vi "test_sample_and_fetch.vi"() -> ()   [LabVIEW 2013, in "varilib.lvlib"]
uses:
  varilib.lvlib
  <instrlib>/niScope/Configure/Trigger/niScope Configure Trigger Immediate.vi
panel:
  in  "status":string
  out "sampling start times":timestamp[](array[timestamp])
  in  "channels (0,1)":string[](array[string])
  in  "generate time axis (T)":bool
  in  "instrument handles":refnum<k15>[](array[refnum])
  out "error out":errorcluster
  out "no of vars in matlab file":i32
  in  "file format (mat)":T1(ring)=enum."csv - semicolon separated values"
  in  "file path and name":path=path "c:/smazat.csv"
  in  "min sample rate":dbl=15000000.0 format="%#_13p"
  in  "min record length":i32=30000000 format="%.0p"
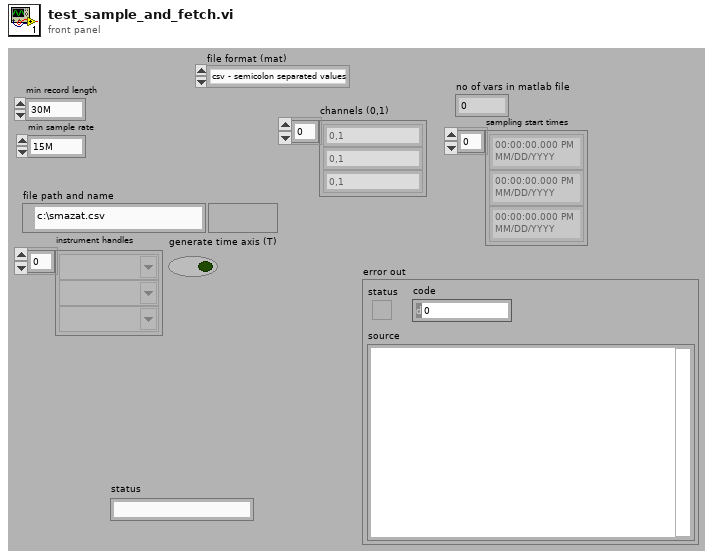
[diagram p1: front panel]
types:
  T1 = enum16{"mat - matlab binary", "csv - semicolon separated values"}
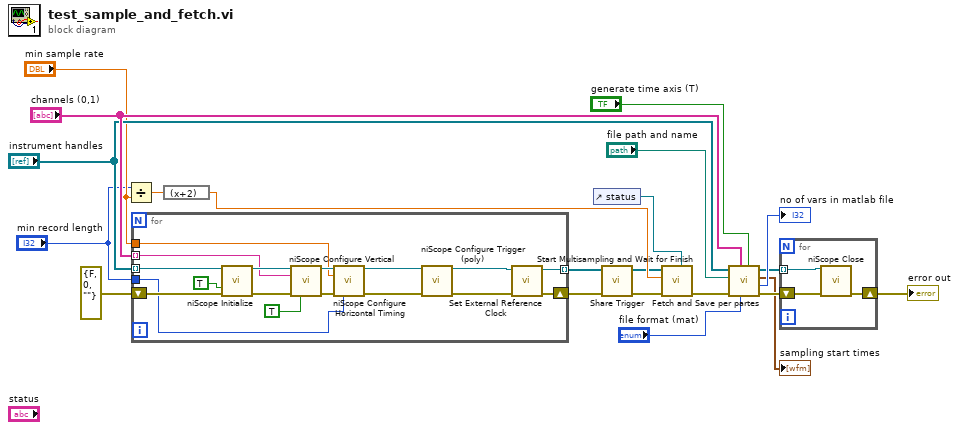
[diagram p0: block diagram]
diagram:
  n1 = Divide(x="min record length", y="min sample rate") -> (x/y=w9:dbl)
  n2 = for {
    tunnel: "channels (0,1)" -> [w30] mode=indexing
    tunnel: "instrument handles" -> [w29] mode=indexing
    shift-right: [w24] -> w3
    shift-left: errorcluster {"status"=FALSE, "code"=0, "source"=""} ("error in") -> [w28]
    tunnel: [w22] -> w4 mode=indexing
    tunnel: "min record length" -> [w27]
    tunnel: "min sample rate" -> [w26]
    n3 = call <instrlib>:"niScope Initialize.vi"("resource name"=w29, "reset device"=TRUE, "error in"=w28) -> ("instrument handle"=w35:refnum<k15>, "error out"=w34:errorcluster)  [unwired: 11 in]
    n4 = call <instrlib>:"niScope Configure Vertical.vi"("instrument handle"=w35, "channels"=w30, "error in"=w34, "channel enabled"=TRUE) -> ("instrument handle out"=w33:refnum<k15>, "error out"=w32:errorcluster)  [unwired: 10 in]
    n5 = call <instrlib>:"niScope Configure Horizontal Timing.vi"("instrument handle"=w33, "min sample rate"=w26, "error in"=w32, "min record length"=w27) -> ("instrument handle out"=w37:refnum<k15>, "error out"=w36:errorcluster)  [unwired: 10 in]
    n6 = call-poly <instrlib>:"niScope Configure Trigger (poly).vi"("instrument handle"=w37, "error in"=w36) -> ("instrument handle out"=w23:refnum<k15>, "error out"=w25:errorcluster)  [unwired: 12 in]
    n7 = call "Set External Reference Clock.vi"("error in (no error)"=w25, "reference"=w23) -> ("error out"=w24:errorcluster, "reference out"=w22:refnum<k15>)  [unwired: 5 in, 3 out]
  }
  n8 = expression code="(x+2)"(w9) -> (w6:dbl)
  n9 = control-ref of="status"() -> (w5:refnum<vi>)
  n10 = call "Share Trigger.vi"("error in"=w3, "instrument handles"=w4) -> ("error out"=w1:errorcluster, "instrument handles out"=w2:refnum<k15>[])  [unwired: 8 in]
  n11 = call "Start Multisampling and Wait for Finish.vi"("status string ref."=w5, "error in"=w1, "timeout"=w6, "instrument handles"=w2) -> ("error out"=w10:errorcluster)  [unwired: 5 in, 2 out]
  n12 = call "Fetch and Save per partes.vi"("generate time axis (T)"="generate time axis (T)", "file format (mat)"="file format (mat)", "channels"="channels (0,1)", "error in"=w10, "file path and name"="file path and name", "instrument handles"="instrument handles") -> ("error out"=w16:errorcluster, "no of vars in matlab file"=→"no of vars in matlab file":i32, "sampling start times"=→"sampling start times":timestamp[], "instrument handles out"=w17:refnum<k15>[])  [unwired: 2 in]
  n13 = for {
    tunnel: w17 -> [w41] mode=indexing
    shift-right: [w39] -> w15
    shift-left: w16 -> [w40]
    n14 = call <instrlib>:"niScope Close.vi"("instrument handle"=w41, "error in"=w40) -> ("error out"=w39:errorcluster)  [unwired: 13 in]
  }
  "error out" <- w15
